vi "Serialize - Text.vi"(8 "error in":errorcluster, 11 "Single_Array in":refnum<class "Single_Array.lvclass">) -> (0 "error out":errorcluster, 2 "Serialized Text":string, 3 "Single_Array out":refnum<class "Single_Array.lvclass">)   [LabVIEW 2016, in "Base Data Class.lvlib" / "Single_Array.lvclass"]
uses:
  Single_Array.lvclass
  Single_Array.lvclass/Single_Array.ctl
  Data.lvclass
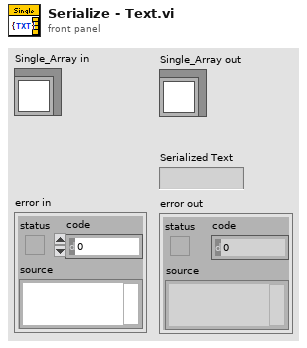
[diagram p1: front panel]
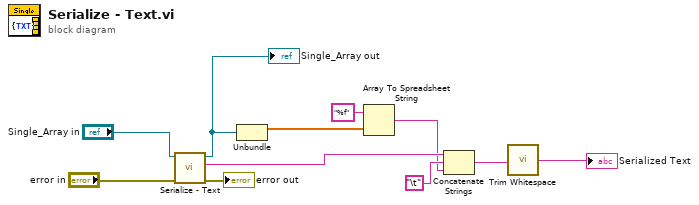
[diagram p0: block diagram]
diagram:
  n1 = call-parent "Serialize - Text.vi"("error in"="error in", "Data in"="Single_Array in") -> ("error out"=→"error out":errorcluster, "Serialized Text"=w5:string, "Data out"=w8:refnum<class "Single_Array.lvclass">)  [unwired: 7 in]
  "Single_Array out" <- w8
  n2 = Unbundle(w8) -> (w7:sgl[])  [unwired: 1 out]
  n3 = Array To Spreadsheet String(array=w7, 3:"%f" ("format string")) -> (spreadsheet string=w3:string)  [unwired: 1 in]
  n4 = Concatenate Strings(w5, "\t", w3) -> (w2:string)
  n5 = call <vilib>:"Trim Whitespace.vi"("string"=w2) -> ("trimmed string"=→"Serialized Text":string)  [unwired: 1 in]
